vi "Write Active Channels.vi"(8 "error in (no error)":errorcluster, 10 "Active Channels":refnum<class "Generic Hardware.lvclass">[](array[class]), 11 "Hardware Settings in":refnum<class "Hardware Settings.lvclass">) -> (0 "error out":errorcluster, 3 "Hardware Settings out":refnum<class "Hardware Settings.lvclass">)   [LabVIEW 2017, in "Hardware Settings.lvclass"]
uses:
  Hardware Settings.lvclass
  Hardware Types/Generic/Generic Hardware.lvclass
  Hardware Settings.lvclass/Hardware Settings.ctl
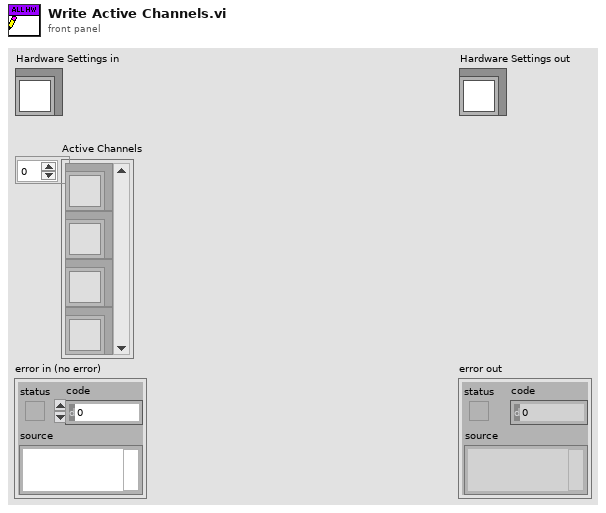
[diagram p1: front panel]
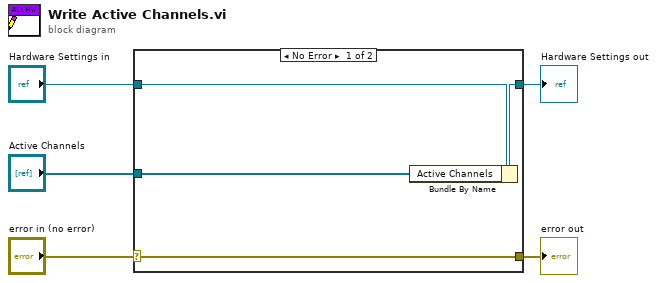
[diagram p0: block diagram]
diagram:
  n1 = case shown="No Error" "error in (no error)" {
    selector: "error in (no error)" -> [w9 w10]
    tunnel: [w9 w10] -> w4
    tunnel: [w7 w11] -> w2
    tunnel: "Hardware Settings in" -> [w8 w11]
    tunnel: "Active Channels" -> [w6 _]
    frame No Error {
      n2 = Bundle By Name(cluster=w8, "Active Channels"=w6) -> (w7:refnum<class "Hardware Settings.lvclass">)
    }
    frame Error {
    }
  }
  "error out" <- w4
  "Hardware Settings out" <- w2
